vi "23-1.vi"() -> ()   [LabVIEW 2019, in "23.lvlib"]
uses:
  23.lvlib
  Burrow/Burrow.lvclass
  Amphipod/Amphipod.lvclass
panel:
  out "Moves List":string[](array[string])
  in  "Sample?":bool
  in  "Sample Index":i32
  out "min energy":u64
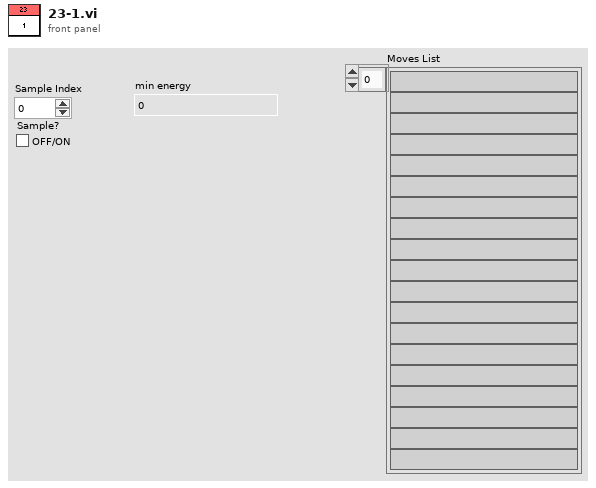
[diagram p1: front panel]
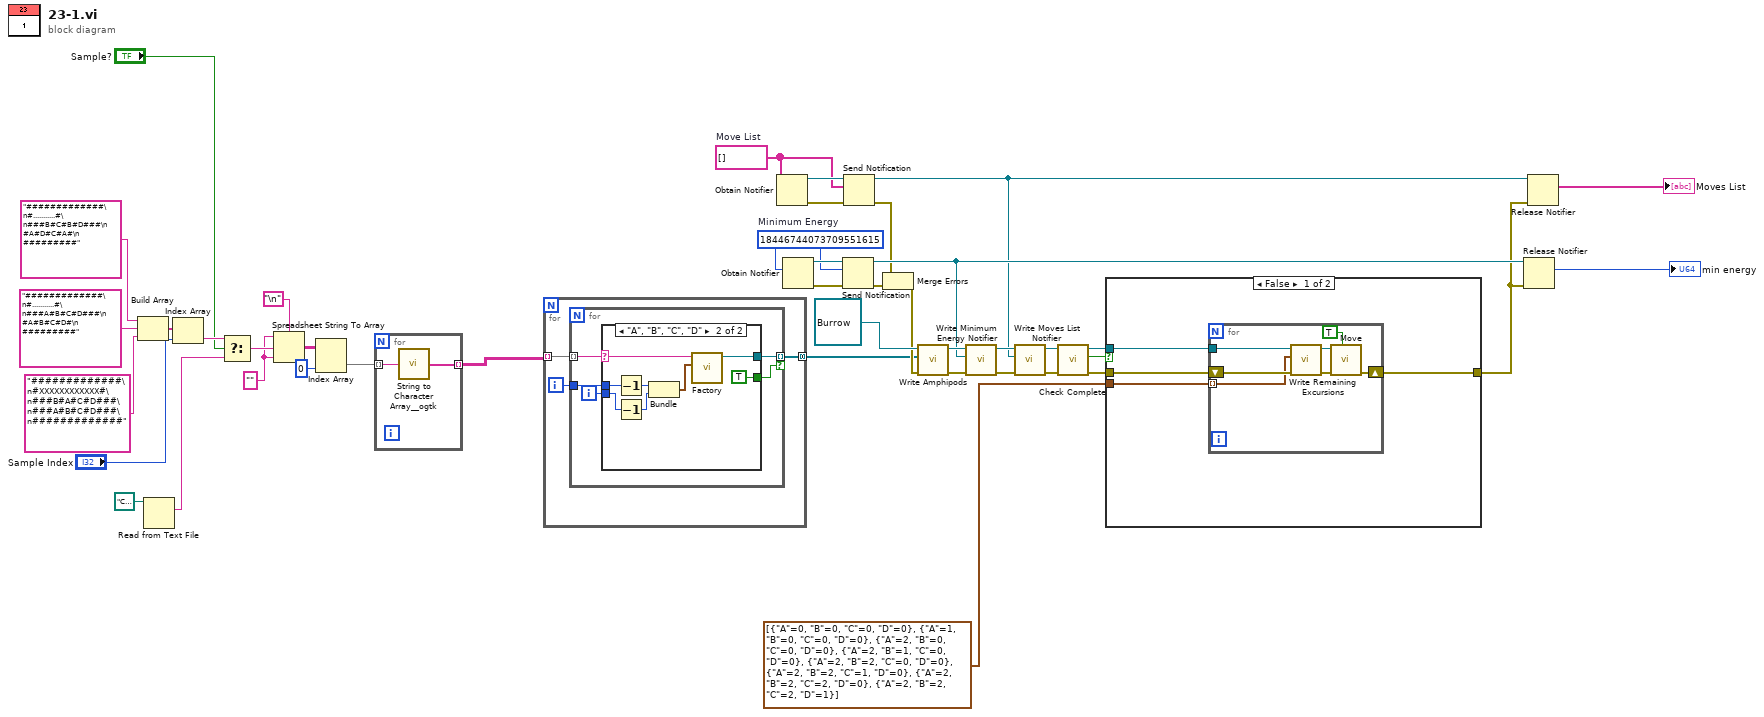
[diagram p0: block diagram]
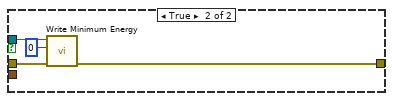
[diagram p3: hidden frame]
diagram:
  w8 = "" ("format string")
  w20 = string[] []  # Move List
  w30 = u64 18446744073709551615  # Minimum Energy
  n1 = Build Array("#############\n#...........#\n###B#C#B#D###\n  #A#D#C#A#\n  #########", "#############\n#...........#\n###A#B#C#D###\n  #A#B#C#D#\n  #########", "#############\n#XXXXXXXXXXXX#\n###B#A#C#D###\n###A#B#C#D###\n#############") -> (w40:string[])
  n2 = Read from Text File(file (use dialog)=path "C:/Users/craig.walker/Documents/GitHub/lv2019-Advent-of-Code-2021/23/input.txt") -> (text=w35:string)  [unwired: 3 in, 3 out]
  n3 = Index Array(array=w40, index="Sample Index") -> (element=w36:string)
  n4 = Select(t=w36, s="Sample?", f=w35) -> (s? t:f=w9:string)
  n5 = Spreadsheet String To Array(delimiter (Tab)="\n", format string=w8, spreadsheet string=w9, array type (2D Dbl)=w8) -> (array=w6:string[][])
  n6 = Index Array(array=w6, index (col)=0 ("disabled index (col)")) -> (element=w4:string[])  [unwired: 1 in]
  n7 = for {
    tunnel: w4 -> [w44] mode=indexing
    tunnel: [w43] -> w5 mode=indexing
    n8 = call <userlib>:"String to Character Array__ogtk.vi"("Input String"=w44) -> ("Character Array"=w43:string[])
  }
  n9 = for {
    tunnel: w5 -> [w47] mode=indexing
    tunnel: [w45] -> w1 mode=concatenating
    i -> [w46]
    n10 = for {
      tunnel: w47 -> [w52] mode=indexing
      tunnel: w46 -> [w51]
      tunnel: [w49] -> w45 mode=indexing if=w48
      i -> [w50]
      n11 = case shown="\"A\", \"B\", \"C\", \"D\"" w52 {
        selector: w52 -> [_ w60]
        tunnel: w51 -> [_ w59]
        tunnel: w50 -> [_ w57]
        tunnel: [_ w55] -> w49
        tunnel: [_ TRUE] -> w48
        frame "False", Default {
        }
        frame "A", "B", "C", "D" {
          n12 = Decrement(x=w59) -> (x-1=w53:i32)
          n13 = Decrement(x=w57) -> (x-1=w56:i32)
          n14 = Bundle(w53, w56) -> (w58:cluster{i32, i32})  [unwired: 1 in]
          n15 = call "Factory.vi"("Position"=w58, "Type"=w60) -> ("Amphipod"=w55:refnum<class "Amphipod.lvclass">)  [unwired: 8 in, 1 out]
        }
      }
    }
  }
  n16 = Obtain Notifier(notification data type=w20) -> (notifier out=w21:refnum<notifier>, error out=w19:errorcluster)  [unwired: 3 in, 1 out]
  n17 = Obtain Notifier(notification data type=w30) -> (notifier out=w32:refnum<notifier>, error out=w31:errorcluster)  [unwired: 3 in, 1 out]
  n18 = Send Notification(notification=w30, notifier=w32, error in (no error)=w31) -> (notifier out=w26:refnum<notifier>, error out=w27:errorcluster)
  n19 = Send Notification(notification=w20, notifier=w21, error in (no error)=w19) -> (notifier out=w10:refnum<notifier>, error out=w15:errorcluster)
  n20 = Merge Errors(w15, w27) -> (w16:errorcluster)
  n21 = call-dynamic "Write Amphipods.vi"("error in (no error)"=w16, "Amphipods"=w1, "Burrow in"=refnum<class "Burrow.lvclass"> refnum) -> ("error out"=w29:errorcluster, "Burrow out"=w28:refnum<class "Burrow.lvclass">)  [unwired: 7 in]
  n22 = call-dynamic "Write Minimum Energy Notifier.vi"("error in (no error)"=w29, "Minimum Energy Notifier"=w26, "Burrow in"=w28) -> ("error out"=w12:errorcluster, "Burrow out"=w14:refnum<class "Burrow.lvclass">)  [unwired: 7 in]
  n23 = call-dynamic "Write Moves List Notifier.vi"("error in (no error)"=w12, "Moves List Notifier"=w10, "Burrow in"=w14) -> ("error out"=w11:errorcluster, "Burrow out"=w13:refnum<class "Burrow.lvclass">)  [unwired: 7 in]
  n24 = call-dynamic "Check Complete.vi"("error in (no error)"=w11, "Burrow in"=w13) -> ("error out"=w23:errorcluster, "Complete?"=w22:bool, "Burrow out"=w24:refnum<class "Burrow.lvclass">)  [unwired: 7 in]
  n25 = case shown="False" w22 {
    tunnel: [w64 w72] -> w17
    tunnel: w24 -> [w63 w75]
    tunnel: w23 -> [w62 w74]
    tunnel: cluster{"A":u8, "B":u8, "C":u8, "D":u8}[] [{"A"=0, "B"=0, "C"=0, "D"=0}, {"A"=1, "B"=0, "C"=0, "D"=0}, {"A"=2, "B"=0, "C"=0, "D"=0}, {"A"=2, "B"=1, "C"=0, "D"=0}, {"A"=2, "B"=2, "C"=0, "D"=0}, {"A"=2, "B"=2, "C"=1, "D"=0}, {"A"=2, "B"=2, "C"=2, "D"=0}, {"A"=2, "B"=2, "C"=2, "D"=1}] ("Remaining Excursions") -> [w61 _]
    frame False {
      n26 = for {
        tunnel: w63 -> [w67]
        shift-right: [w71] -> w64
        shift-left: w62 -> [w70]
        tunnel: w61 -> [w66] mode=indexing
        n27 = call-dynamic "Write Remaining Excursions.vi"("error in (no error)"=w70, "Remaining Excursions"=w66, "Burrow in"=w67) -> ("error out"=w69:errorcluster, "Burrow out"=w68:refnum<class "Burrow.lvclass">)  [unwired: 7 in]
        n28 = call-dynamic "Move.vi"("Part 1"=TRUE, "error in (no error)"=w69, "Burrow in"=w68) -> ("error out"=w71:errorcluster)  [unwired: 8 in]
      }
    }
    frame True {
      n29 = call-dynamic "Write Minimum Energy.vi"("error in (no error)"=w74, "Minimum Energy"=u64 0, "Burrow in"=w75) -> ("error out"=w72:errorcluster)  [unwired: 7 in, 1 out]
    }
  }
  n30 = Release Notifier(notifier=w26, error in (no error)=w17) -> (last notification=→"min energy":u64)  [unwired: 1 in, 2 out]
  n31 = Release Notifier(notifier=w10, error in (no error)=w17) -> (last notification=→"Moves List":string[])  [unwired: 1 in, 2 out]
